vi "SetDataType.vi"(0 "object in":refnum<class "Client.lvclass">, 2 "File Type":T1, 5 "Error In":errorcluster) -> (14 "object out":refnum<class "Client.lvclass">, 19 "Error Out":errorcluster)   [LabVIEW 2024, in "Client.lvclass"]
uses:
  Client.lvclass
  Support/Type Def/File Type.ctl
  Abstractions/TDMS/TDMS.lvclass
  C:/Users/burakkorkmaz/Desktop/Leveling/labview-desing-patterns/Bridge Pattern/Abstractions/DataType/DataType.lvclass
  Abstractions/Excel/Excel.lvclass
  Client.lvclass/Client.ctl
  Abstractions/DataType/DataType.lvclass
  <vilib>/Utility/file.llb/Write Delimited Spreadsheet (string).vi
panel:
  # "Connector Pane"
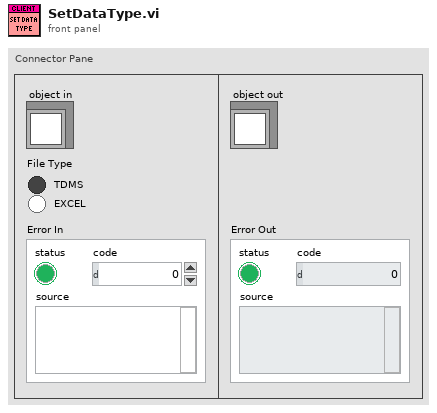
[diagram p1: front panel]
types:
  T1 = typedef "File Type.ctl" = enum32{"TDMS", "EXCEL"}
  T2 = enum16{"open", "open or create", "create or replace", "create", "open (read-only)"}
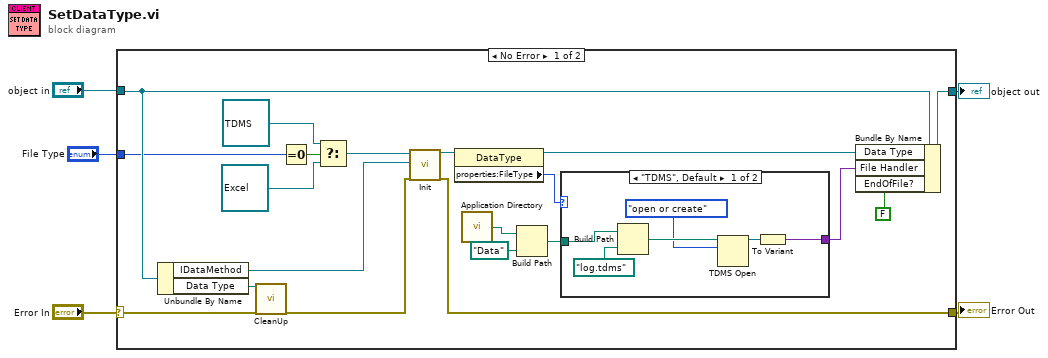
[diagram p0: block diagram]
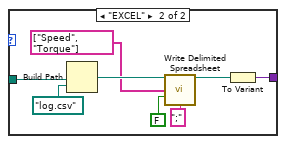
[diagram p2: hidden frame]
diagram:
  n1 = case shown="No Error" "Error In" {
    selector: "Error In" -> [w22 w41]
    tunnel: [w14 w41] -> w4
    tunnel: [w25 w40] -> w2
    tunnel: "object in" -> [w24 w40]
    tunnel: "File Type" -> [w20 _]
    frame No Error {
      n2 = Unbundle By Name(w24) -> ("IDataMethod"=w13:refnum<class "IDataMethod.lvclass">, "Data Type"=w23:refnum<class "DataType.lvclass">)
      n3 = call-dynamic "CleanUp.vi"("object in"=w23, "error in (no error)"=w22) -> ("error out"=w15:errorcluster)  [unwired: 16 in, 1 out]
      n4 = Equal To 0?(x=w20) -> (x = 0?=w21:bool)
      n5 = Select(t=refnum<class "TDMS.lvclass"> refnum ("TDMS"), s=w21, f=refnum<class "Excel.lvclass"> refnum ("Excel")) -> (s? t:f=w17:refnum<class "DataType.lvclass">)
      n6 = call-dynamic "Init.vi"("object in"=w17, "Data Method"=w13, "error in (no error)"=w15) -> ("object out"=w16:refnum<class "DataType.lvclass">, "error out"=w14:errorcluster)  [unwired: 15 in]
      n7 = property class="DataType"(reference=w16) -> (reference out=w9:refnum<class "DataType.lvclass">, "properties:FileType"=w8:T1)  [unwired: 1 in, 1 out]
      n8 = call <vilib>:"Application Directory.vi"() -> ("Application Directory"=w10:path)
      n9 = Build Path(base path=w10, name or relative path=path "Data") -> (appended path=w12:path)
      n10 = case shown="\"TDMS\", Default" w8 {
        tunnel: w12 -> [w31 w38]
        tunnel: [w26 w32] -> w7
        frame "TDMS", Default {
          n11 = Build Path(base path=w31, name or relative path=path "log.tdms") -> (appended path=w30:path)
          n12 = TDMS Open(10:T2."open or create" ("operation (0:open)"), 11:w30) -> (3:w27:refnum<k34>)  [unwired: 5 in, 1 out]
          n13 = To Variant(anything=w27) -> (Variant=w26:variant)
        }
        frame "EXCEL" {
          n14 = Build Path(base path=w38, name or relative path=path "log.csv") -> (appended path=w36:path)
          n15 = call-poly <vilib>:"Write Delimited Spreadsheet.vi"("file path (dialog if empty)"=w36, "1D data"=string[] ["Speed", "Torque"], "append to file? (new file:F)"=FALSE, "delimiter (\\t)"=";" ("delimiter (\\t)")) -> ("new file path (Not A Path if cancelled)"=w39:path)  [unwired: 10 in, 1 out]
          n16 = To Variant(anything=w39) -> (Variant=w32:variant)
        }
      }
      n17 = Bundle By Name(cluster=w24, "Data Type"=w9, "File Handler"=w7, "EndOfFile?"=FALSE) -> (w25:refnum<class "Client.lvclass">)
    }
    frame Error {
    }
  }
  "Error Out" <- w4
  "object out" <- w2
